vi "Example 6 (Import All Scalars).vi"() -> ()   [LabVIEW 2018]
uses:
  <vilib>/addons/VeriStand Custom Device Scripting APIs/FPGA Addon/Scripting API.lvlibp/APIs/Scripting API/TypeDefs/Output Scalar Data.ctl
  <vilib>/addons/VeriStand Custom Device Scripting APIs/FPGA Addon/Scripting API.lvlibp/Addon/Addon Shared/Types/Data Type.ctl
  <vilib>/addons/VeriStand Custom Device Scripting APIs/FPGA Addon/Scripting API.lvlibp/APIs/Scripting API/Public/Bitfile Resources/Import Bitfile Scalars (Instances)/Import Scalars - all.vi
  <vilib>/addons/VeriStand Custom Device Scripting APIs/FPGA Addon/Scripting API.lvlibp
  <vilib>/addons/VeriStand Custom Device Scripting APIs/FPGA Addon/Scripting API.lvlibp/Addon/Addon Shared/FPGA Addon Shared.lvlib
panel:
  out "size(s)":i32
  out "bitfile scalars out":T1[](array[typedef])
  out "error out":errorcluster
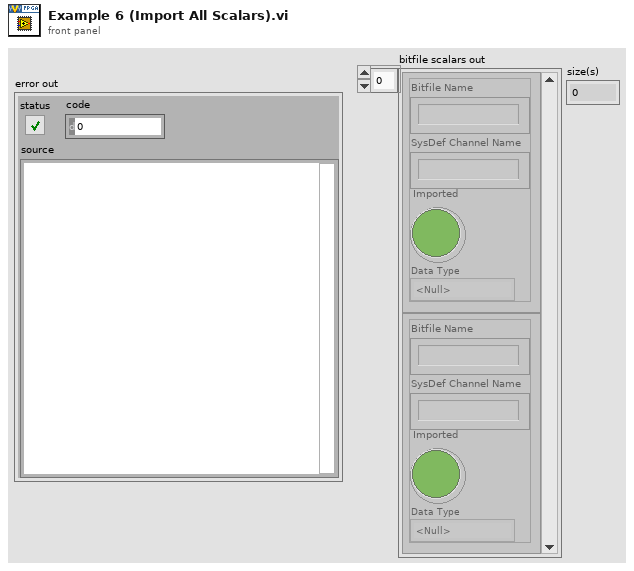
[diagram p1: front panel]
types:
  T1 = typedef "Scripting API.lvlibp/Output Scalar Data.ctl" = cluster{"Bitfile Name":string, "SysDef Channel Name":string, "Imported":bool, "Data Type":T2}
  T2 = typedef "Scripting API.lvlibp/FPGA Addon Shared.lvlib/Data Type.ctl" = enum8{"<Null>", "I8", "I16", "I32", "I64", "U8", "U16", "U32", "U64", "SGL", "Boolean", "Analog PWM In Settings", "Analog PWM In", "Digital PWM In Settings", "Digital PWM In", "Digital PWM Out", "Sine Out", "FXP+/-24.5", "FXP+/-16.5", "FXP+/-32.8", "FXP+/-64.32", "FXP+/-16.7", "FXP+/-20.5", "FXP+/-27.5", "FXP+/-32.16", "FXP+16.3", "FXP+18.3", "Digital Static In", "Digital Static Out", "Digital Static In Settings", "Digital WSS Out", "Quad Encoder Settings", "Quad Encoder In", "Group"}
  T3 = typedef "Scripting API.lvlibp/Custom Device API.lvlib/Custom Device Item Ref.ctl" = u64
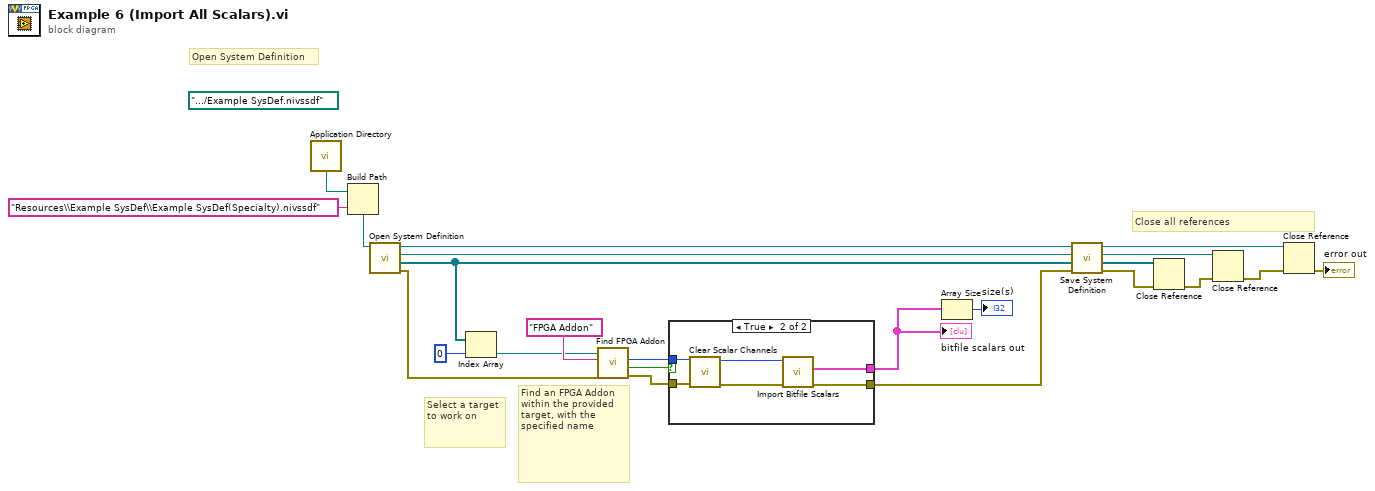
[diagram p0: block diagram]
diagram:
  (unwired) path ".../Example SysDef.nivssdf" ("fpga bitfile path")
  # "Close all references"
  # "Find an FPGA Addon within the provided target, with the specified name"
  # "Select a target to work on"
  # "Open System Definition"
  n1 = call <vilib>:"Application Directory.vi"() -> ("Application Directory"=w16:path)
  n2 = Build Path(base path=w16, name or relative path="Resources\\Example SysDef\\Example SysDef(Specialty).nivssdf") -> (appended path=w14:path)
  n3 = call "Open System Definition.vi"("System Definition File"=w14) -> ("error out"=w4:errorcluster, "targets refnums"=w19:refnum<k24>[], "root refnum"=w20:refnum<k24>, "system definition refnum"=w12:refnum<k24>)  [unwired: 7 in]
  n4 = Index Array(array=w19, index=0) -> (element=w5:refnum<k24>)
  n5 = call <vilib>:"Find FPGA Addon.vi"("error in (no error)"=w4, "FPGA Addon name"="FPGA Addon" ("fpga addon name"), "target in"=w5) -> ("error out"=w7:errorcluster, "found ?"=w6:bool, "FPGA Addon refnum out"=w8:T3)  [unwired: 5 in, 1 out]
  n6 = case shown="True" w6 {
    tunnel: w8 -> [_ w28]
    tunnel: w7 -> [w22 w27]
    tunnel: [_ w24] -> w2
    tunnel: [w22 w23] -> w1
    frame False {
    }
    frame True {
      n7 = call <vilib>:"Clear Scalar Channels.vi"("error in (no error)"=w27, "FPGA Addon refnum in"=w28) -> ("error out"=w25:errorcluster, "FPGA Addon refnum out"=w26:T3)  [unwired: 8 in]
      n8 = call-poly <vilib>:"Import Bitfile Scalars.vi"("error in (no error)"=w25, "FPGA Addon refnum in"=w26) -> ("error out"=w23:errorcluster, "imported bitfile scalars out"=w24:T1[])  [unwired: 7 in, 1 out]
    }
  }
  "bitfile scalars out" <- w2
  n9 = Array Size(array=w2) -> (size(s)=→"size(s)":i32)
  n10 = call "Save System Definition.vi"("error in (no error)"=w1, ".NET Refnum in"=w12) -> ("error out"=w10:errorcluster, ".NET Refnum out"=w11:refnum<k24>)  [unwired: 8 in]
  n11 = Close Reference(reference=w19, error in (no error)=w10) -> (error out=w18:errorcluster)
  n12 = Close Reference(reference=w20, error in (no error)=w18) -> (error out=w17:errorcluster)
  n13 = Close Reference(reference=w11, error in (no error)=w17) -> (error out=→"error out":errorcluster)
